vi "Create Instance Impl.vi"(8 "error in (no error)":errorcluster, 10 "Stage Configuration":T1={"Serial Port"="COM4", "Forward Step (mm)"=0.4, "Lane Length (mm)"=6.0, "Lane Separation (mm)"=0.8, "Stage Type"=enum."Ti2", "Autofocus Z Planes"=9, "Autofocus Range (um)"=30.0, "Stage Limits"={"Y Min"=-4.5, "Y Max"=3.0, "X Min"=-19.0, "X Max"=33.5}, "Slide (mm)"={"top"=-13.0, "right"=-22.3, "width"=60.0, "height"=25.4}}, 11 "Newport ESP301 Stage in":refnum<class "Newport ESP301 Stage.lvclass">) -> (0 "error out":errorcluster, 3 "Newport ESP301 Stage out":refnum<class "Newport ESP301 Stage.lvclass">)   [LabVIEW 2023, in "Newport ESP301 Stage.lvlib" / "Newport ESP301 Stage.lvclass"]
uses:
  Newport ESP301 Stage.lvclass
  Newport ESP301 Stage.lvclass/Newport ESP301 Stage.ctl
  <vilib>/Instr/_visa.llb/VISA Configure Serial Port (Instr).vi
  Resources/Type Defs/Stage Configuration.ctl
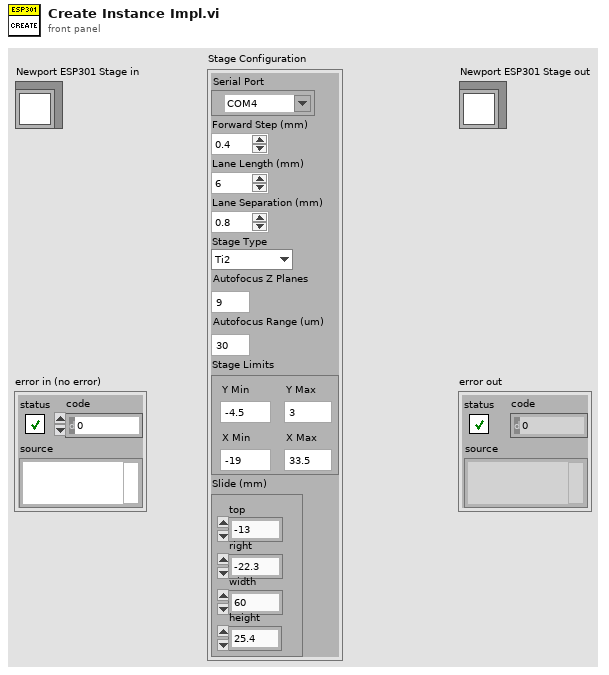
[diagram p1: front panel]
types:
  T1 = typedef "Stage Configuration.ctl" = cluster{"Serial Port":refnum<visa-resource-name>, "Forward Step (mm)":dbl, "Lane Length (mm)":dbl, "Lane Separation (mm)":dbl, "Stage Type":enum16{"Disabled", "ESP301", "Ti2", "Ludl", "ASI"}, "Autofocus Z Planes":i32, "Autofocus Range (um)":dbl, "Stage Limits":cluster{"Y Min":dbl, "Y Max":dbl, "X Min":dbl, "X Max":dbl}, "Slide (mm)":cluster{"top":dbl, "right":dbl, "width":dbl, "height":dbl}}
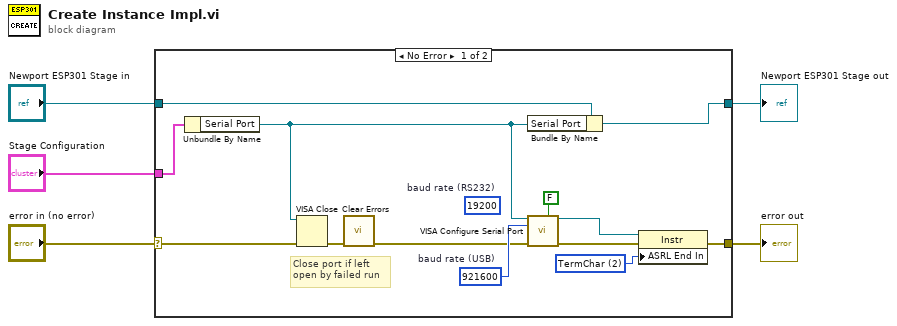
[diagram p0: block diagram]
diagram:
  n1 = case shown="No Error" "error in (no error)" {
    selector: "error in (no error)" -> [w11 w19]
    tunnel: [w8 w19] -> w4
    tunnel: "Newport ESP301 Stage in" -> [w18 w20]
    tunnel: [w17 w20] -> w2
    tunnel: "Stage Configuration" -> [w16 _]
    frame No Error {
      w6 = u16 2 items=["None", "Last Bit", "TermChar"] ("Serial Settings:End Mode for Reads")
      w14 = u32 921600  # baud rate (USB)
      (unwired) u32 19200  # baud rate (RS232)
      # "Close port if left\nopen by failed run"
      n2 = Unbundle By Name(w16) -> ("Serial Port"=w13:refnum<visa-resource-name>)
      n3 = VISA Close(VISA resource name=w13, error in (no error)=w11) -> (error out=w12:errorcluster)
      n4 = call <vilib>:"Clear Errors.vi"("error in (no error)"=w12) -> ("error out"=w10:errorcluster)  [unwired: 5 in, 1 out]
      n5 = Bundle By Name(cluster=w18, "Serial Port"=w13) -> (w17:refnum<class "Newport ESP301 Stage.lvclass">)
      n6 = call-poly "VISA Configure Serial Port"("VISA resource name"=w13, "Enable Termination\nChar (T)"=FALSE ("Enable Termination\nChar (T)"), "baud rate (9600)"=w14, "error in (no error)"=w10) -> ("VISA resource name out"=w7:refnum<visa-resource-name>, "error out"=w9:errorcluster)  [unwired: 10 in]
      n7 = property class="Instr"(reference=w7, error in=w9, "ASRL End In"=w6) -> (error out=w8:errorcluster)  [unwired: 1 out]
    }
    frame Error {
    }
  }
  "error out" <- w4
  "Newport ESP301 Stage out" <- w2
